vi "RDS Child Receive Message.vi"(8 "error in (no error)":errorcluster, 10 "RDS Message":refnum<class "RDS Message.lvclass">, 11 "RDS Helm Actor in":refnum<class "RDS Helm Actor.lvclass">) -> (0 "error out":errorcluster, 3 "RDS Helm Actor out":refnum<class "RDS Helm Actor.lvclass">)   [LabVIEW 2015, in "RDS Helm Actor.lvlib" / "RDS Helm Actor.lvclass"]
uses:
  RDS Helm Actor.lvclass
  Libraries/RDS Framework/RDS Message Class/RDS Message.lvclass
  Libraries/RDS Framework/RDS Message Class/RDS Message.lvclass/RDS Message.ctl
  Libraries/RDS Child Messages/Helm/Heading Command/Heading Command Msg.lvclass
  Helm State.ctl
  Libraries/RDS Child Messages/Helm/Heading Command/Heading Command Msg.lvclass/Heading Command Msg.ctl
  RDS Helm Actor.lvclass/RDS Helm Actor.ctl
  Libraries/RDS Child Messages/Helm/Steering Command/Steering Command.lvclass
  Libraries/RDS Child Messages/Helm/Steering Command/Steering Command.lvclass/Steering Command.ctl
  Libraries/RDS Child Messages/Compass/Compass Data Message.lvclass
  Libraries/RDS Child Messages/Compass/Compass Data Message.lvclass/Compass Data Message.ctl
  Libraries/RDS Child Messages/Helm/Helm Limiter Message/Helm Limiter Msg.lvclass
  Libraries/RDS Child Messages/Helm/Helm Limiter Message/Helm Limiter Msg.lvclass/Helm Limiter Msg.ctl
  Libraries/RDS Child Messages/PID Gains/PID Gains Set Message.lvclass
  Libraries/RDS Child Messages/PID Gains/PID Gains Set Message.lvclass/PID Gains Set Message.ctl
  RDS Helm Actor.lvlib
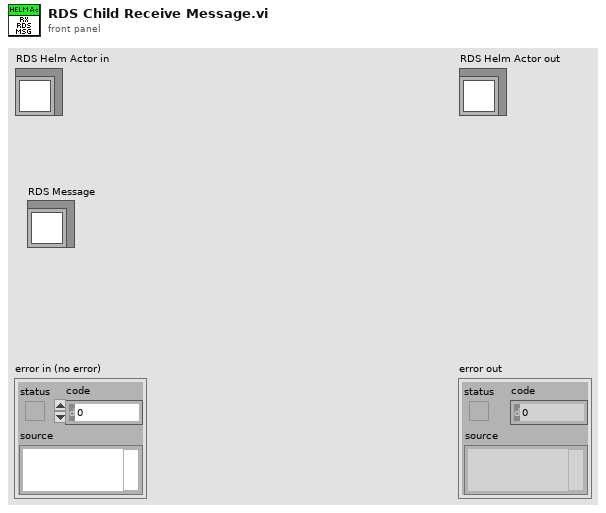
[diagram p1: front panel]
types:
  T1 = typedef "RDS Child Messages.lvlib/RDS Message ID.ctl" = enum16{"RDS Hello World", "String Message", "AIP_Status", "AIP_Command", "GPS_Data", "MCB_Command", "MCB_Status", "Compass_Data", "Depth_Data", "Battery_Data", "Contoller_State", "Set_Mag_Dev", "BTB_Shutdown", "State_Sample_Request", "State_Sample", "PID_Gains_Set", "Helm_Limiter_Set", "Helm_Heading_Command", "Helm_Steering_Command", "Helm_Status", "Controller_Message", "AIP_Set_Min_Depth", "Mission_Controller_State", "Mission_Upload", "Mission_Set_Op_and_Run", "Mission_Settings_Set"}
  T2 = typedef "RDS Helm Actor.lvlib/Helm State.ctl" = enum16{"Idle", "Executing Heading Command", "Executing Steering Command"}
  T3 = typedef "RDS Child Messages.lvlib/Heading Command Cntrl.ctl" = cluster{"Throttle":i16, "Heading":sgl, "Duration (s)":i16}
  T4 = typedef "RDS Child Messages.lvlib/Steering Command Cntrl.ctl" = cluster{"Throttle":i16, "Rudder":i8, "Duration (s)":u16}
  T5 = typedef "RDS Instrument Library.lvlib/Compass Data.ctl" = cluster{"Compass Heading":sgl, "pitch Angle":sgl, "roll Angle":sgl, "Temperature":sgl, "Depth":sgl, "Magnetic Field":sgl, "Magnetic Field X":sgl, "Magnetic Field Y":sgl, "Magnetic Field Z":sgl, "Acceleration":sgl, "Acceleration X":sgl, "Acceleration Y":sgl, "Gyro":sgl, "Gyro X":sgl, "Acceleration Z":sgl, "Gyro Y":sgl, "Raw Heading":sgl}
  T6 = typedef "RDS Child Messages.lvlib/PID Gains Control.ctl" = cluster{"P (Kc)":sgl, "I (Ti)":sgl, "D (Td)":sgl}
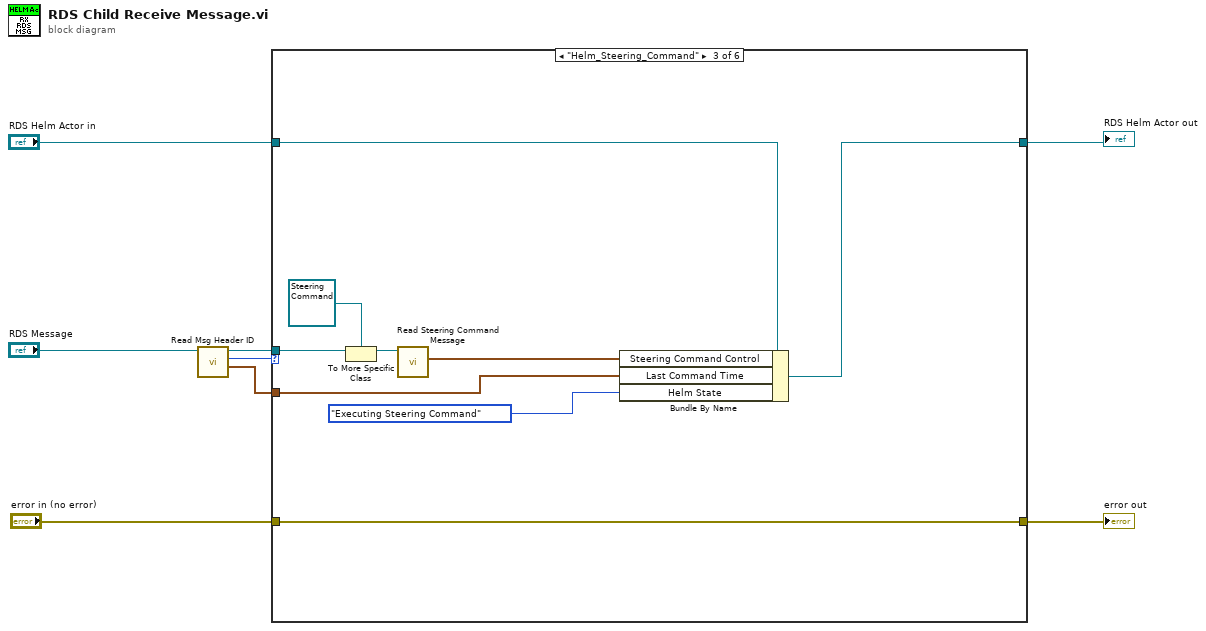
[diagram p0: block diagram]
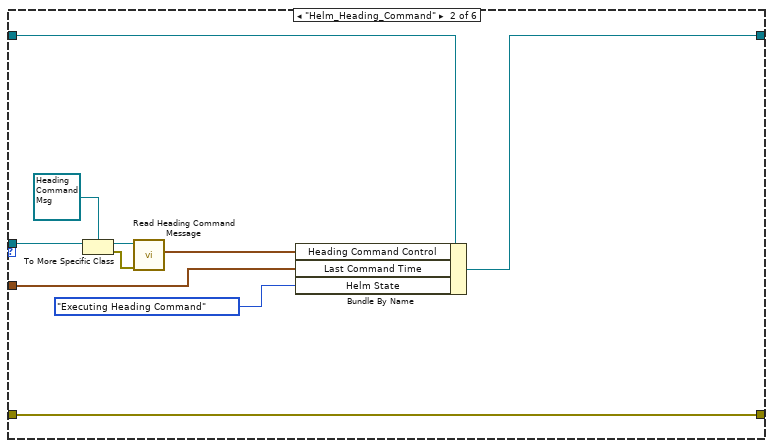
[diagram p3: hidden frame]
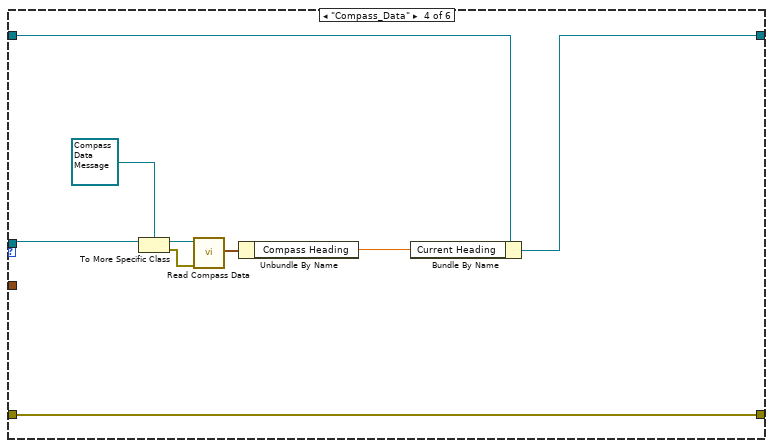
[diagram p4: hidden frame]
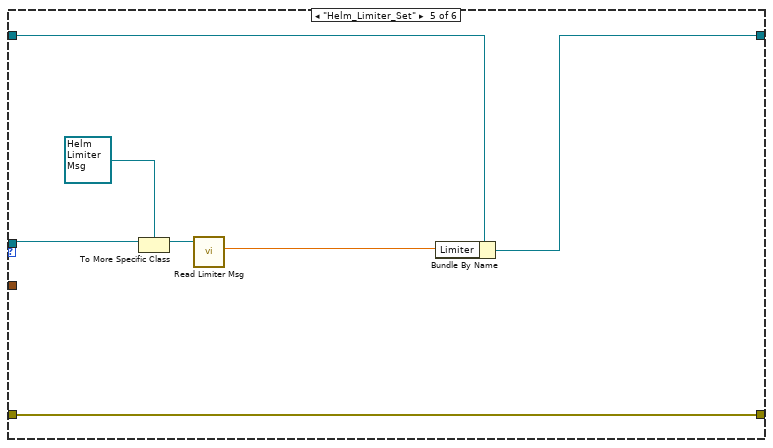
[diagram p5: hidden frame]
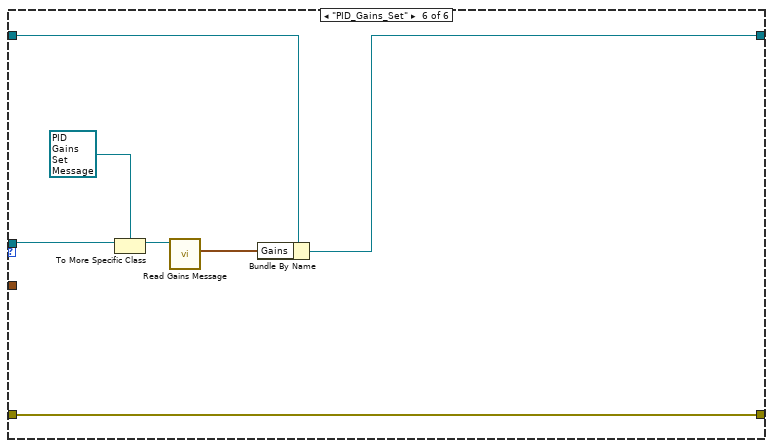
[diagram p6: hidden frame]
diagram:
  n1 = call "Read Msg Header ID.vi"("RDS Message in"="RDS Message") -> ("Time Stamp"=w1:timestamp, "Msg ID"=w8:T1, "RDS Message out"=w7:refnum<class "RDS Message.lvclass">)  [unwired: 6 in, 2 out]
  n2 = case shown="\"Helm_Steering_Command\"" w8 {
    tunnel: "RDS Helm Actor in" -> [w9 w16 w28 w32 w44 w49]
    tunnel: [w10 w12 w22 w30 w42 w46] -> w3
    tunnel: "error in (no error)" -> [w10 w12 w22 w30 w42 w46]
    tunnel: w7 -> [_ w20 w29 w38 w45 w51]
    tunnel: [w9 w13 w26 w31 w43 w47] -> w2
    tunnel: w1 -> [_ w14 w27 _ _ _]
    frame "RDS Hello World", Default {
    }
    frame "Helm_Heading_Command" {
      n3 = To More Specific Class(target class=refnum<class "Heading Command Msg.lvclass"> refnum ("RDS Child Messages.lvlib:Heading Command Msg.lvclass"), reference=w20) -> (specific class reference=w17:refnum<class "Heading Command Msg.lvclass">, error out=w18:errorcluster)  [unwired: 1 in]
      n4 = call "Read Heading Command Message.vi"("error in (no error)"=w18, "Heading Command Msg in"=w17) -> ("Heading Command Control"=w15:T3)  [unwired: 7 in, 2 out]
      n5 = Bundle By Name(cluster=w16, "Heading Command Control"=w15, "Last Command Time"=w14, "Helm State"=Helm_State."Executing Heading Command") -> (w13:refnum<class "RDS Helm Actor.lvclass">)
    }
    frame "Helm_Steering_Command" {
      n6 = To More Specific Class(target class=refnum<class "Steering Command.lvclass"> refnum ("RDS Child Messages.lvlib:Steering Command.lvclass"), reference=w29) -> (specific class reference=w24:refnum<class "Steering Command.lvclass">)  [unwired: 1 in, 1 out]
      n7 = call "Read Steering Command Message.vi"("Steering Command in"=w24) -> ("Steering Command Control"=w23:T4)  [unwired: 8 in, 2 out]
      n8 = Bundle By Name(cluster=w28, "Steering Command Control"=w23, "Last Command Time"=w27, "Helm State"=Helm_State."Executing Steering Command") -> (w26:refnum<class "RDS Helm Actor.lvclass">)
    }
    frame "Compass_Data" {
      n9 = To More Specific Class(target class=refnum<class "Compass Data Message.lvclass"> refnum ("RDS Child Messages.lvlib:Compass Data Message.lvclass"), reference=w38) -> (specific class reference=w35:refnum<class "Compass Data Message.lvclass">, error out=w36:errorcluster)  [unwired: 1 in]
      n10 = call "Read Compass Data.vi"("error in (no error)"=w36, "Compass Data Message in"=w35) -> ("Compass Data"=w34:T5)  [unwired: 7 in, 2 out]
      n11 = Unbundle By Name(w34) -> ("Compass Heading"=w33:sgl)
      n12 = Bundle By Name(cluster=w32, "Current Heading"=w33) -> (w31:refnum<class "RDS Helm Actor.lvclass">)
    }
    frame "Helm_Limiter_Set" {
      n13 = To More Specific Class(target class=refnum<class "Helm Limiter Msg.lvclass"> refnum ("RDS Child Messages.lvlib:Helm Limiter Msg.lvclass"), reference=w45) -> (specific class reference=w40:refnum<class "Helm Limiter Msg.lvclass">)  [unwired: 1 in, 1 out]
      n14 = call "Read Limiter Msg.vi"("Helm Limiter Msg in"=w40) -> ("Limiter"=w39:dbl)  [unwired: 8 in, 2 out]
      n15 = Bundle By Name(cluster=w44, "Limiter"=w39) -> (w43:refnum<class "RDS Helm Actor.lvclass">)
    }
    frame "PID_Gains_Set" {
      n16 = To More Specific Class(target class=refnum<class "PID Gains Set Message.lvclass"> refnum ("RDS Child Messages.lvlib:PID Gains Set Message.lvclass"), reference=w51) -> (specific class reference=w50:refnum<class "PID Gains Set Message.lvclass">)  [unwired: 1 in, 1 out]
      n17 = call "Read Gains Message.vi"("PID Gains Set Message in"=w50) -> ("Gains"=w48:T6)  [unwired: 8 in, 2 out]
      n18 = Bundle By Name(cluster=w49, "Gains"=w48) -> (w47:refnum<class "RDS Helm Actor.lvclass">)
    }
  }
  "error out" <- w3
  "RDS Helm Actor out" <- w2
